vi "ChangeFreqWFG.vi"(0 "object in":refnum<class "InstrumentBase.lvclass">, 2 "Freq Ch1&2":T1, 5 "error in (no error)":errorcluster) -> (14 "object out":refnum<class "InstrumentBase.lvclass">, 19 "error out":errorcluster)   [LabVIEW 2019, in "InstrumentBase.lvclass"]
uses:
  InstrumentBase.lvclass
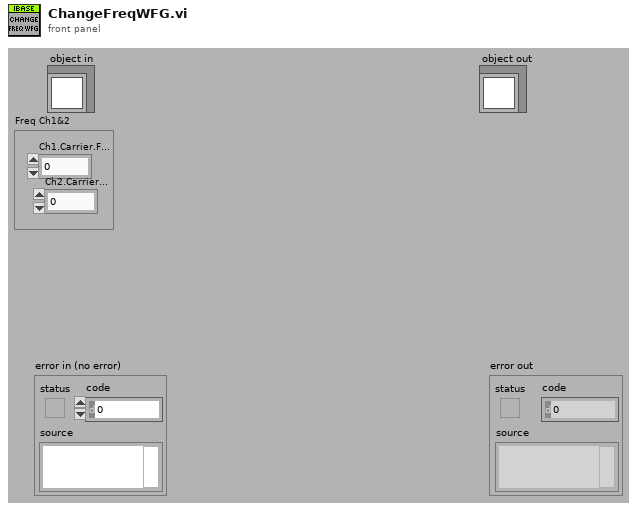
[diagram p1: front panel]
types:
  T1 = cluster{"Ch1.Carrier.Frequency (Hz)":dbl, "Ch2.Carrier.Frequency (Hz)":dbl}
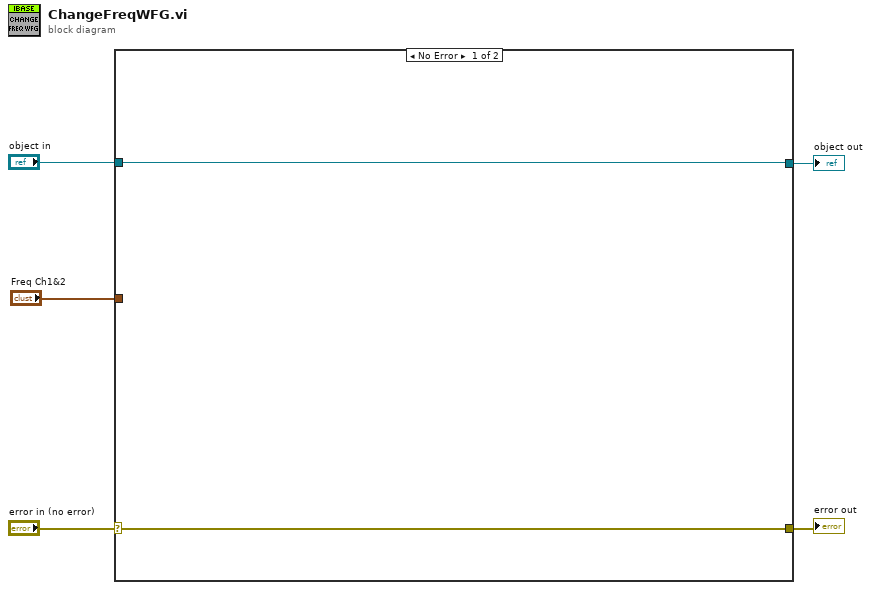
[diagram p0: block diagram]
diagram:
  n1 = case shown="No Error" "error in (no error)" {
    selector: "error in (no error)" -> [w6 w9]
    tunnel: [w6 w9] -> w4
    tunnel: [w7 w8] -> w2
    tunnel: "object in" -> [w7 w8]
    tunnel: "Freq Ch1&2" -> [_ _]
    frame No Error {
    }
    frame Error {
    }
  }
  "error out" <- w4
  "object out" <- w2
